vi "TUNA RT main.vi"() -> ()   [LabVIEW 2014]
uses:
  <vilib>/myRIO/Instrument Drivers/Onboard IO/AI/AI.lvlib
  <vilib>/myRIO/Common/Instrument Driver Framework/Utilities/typedefs/Analog Scaling Constants.ctl
  <vilib>/myRIO/Common/Instrument Driver Framework/Utilities/typedefs/Analog Scaling Constants List.ctl
  <vilib>/myRIO/Common/Instrument Driver Framework/myRIO v1.0/AI/typedefs/AI Channels Enum.ctl
  <vilib>/myRIO/Common/Instrument Driver Framework/myRIO v1.0/AI/typedefs/AI Channels List.ctl
  <vilib>/myRIO/Common/Instrument Driver Framework/Utilities/typedefs/Generic FPGA Reference.ctl
  <vilib>/myRIO/Common/Instrument Driver Framework/Utilities/typedefs/myRIO v1.0 Reference.ctl
  <vilib>/myRIO/Common/Instrument Driver Framework/Utilities/typedefs/Hardware Version Enum.ctl
  <vilib>/myRIO/Common/Instrument Driver Framework/Utilities/typedefs/myRIO Generic Hardware Reference.ctl
  <vilib>/myRIO/Instrument Drivers/Onboard IO/AI/typedefs/AI Reference.ctl
  <vilib>/userdefined/High Color/nirio_resource_hc.ctl
  <vilib>/myRIO/Instrument Drivers/Onboard IO/AI/vis/myRIO AI Open.xnode
  <vilib>/myRIO/Common/Instrument Driver Framework/myRIO v1.0/DIO/typedefs/DIO Channels Enum.ctl
  <vilib>/myRIO/Common/Instrument Driver Framework/myRIO v1.0/DIO/typedefs/DIO Channels List.ctl
  <vilib>/myRIO/Instrument Drivers/Onboard IO/DIO/typedefs/DIO Reference.ctl
  <vilib>/myRIO/Instrument Drivers/Onboard IO/DIO/DIO.lvlib
  <vilib>/myRIO/Instrument Drivers/Onboard IO/DIO/vis/myRIO DIO Open.xnode
  <vilib>/myRIO/Instrument Drivers/Onboard IO/PWM/typedefs/PWM Configuration.ctl
  <vilib>/myRIO/Instrument Drivers/Onboard IO/PWM/PWM.lvlib
  <vilib>/myRIO/Common/Instrument Driver Framework/myRIO v1.0/PWM/typedefs/PWM Channels Enum.ctl
  <vilib>/myRIO/Instrument Drivers/Onboard IO/PWM/typedefs/PWM Reference.ctl
  <vilib>/myRIO/Instrument Drivers/Onboard IO/PWM/vis/myRIO PWM Open.xnode
  <vilib>/myRIO/Common/Instrument Driver Framework/myRIO v1.0/PWM/vis/myRIO v1.1 Open PWM.vi
  <vilib>/myRIO/Common/Instrument Driver Framework/myRIO v1.0/AI/vis/myRIO v1.1 Open AI.vi
  <vilib>/myRIO/Common/Instrument Driver Framework/myRIO v1.0/DIO/vis/myRIO v1.1 Open DIO.vi
  <vilib>/Instr/_visa.llb/VISA Flush IO Buffer Mask.ctl
panel:
  in  "LHEADING":dbl
  in  "LSPEED":dbl
  in  "LTAIL PERIOD":dbl
  in  "Tab Control":T1(tab)
  in  "MHeading":dbl(slide) scale=0.0005..0.0025 scale format="%_1f"
  in  "MSpeed":dbl(slide) scale=0.0005..0.0025 scale format="%#.1g"
  out "GLED":bool
  out "BLED":bool
  out "RLED":bool
  in  "stop":bool
  out "Midbrain?":bool
  out "Heading":dbl(knob) min=-45.0 max=45.0 step=1.0 scale=-45.0..45.0
  out "Speed":dbl(knob) min=-9.0 max=9.0 step=1.0 scale=-50.0..50.0
  out "Hindbrain?":bool
  out "Forebrain?":bool
  out "Battery Dead?":bool
  out "Complete?":bool=TRUE
  out "Arbiter Graph":cluster{dbl, dbl, dbl[]}(graph)
  out "GPS Time Out?":bool
  in  "Run?":bool
  in  "Manual?":bool
  out "Camera Data":T2(array[cluster])
  out "Boat Status":T3={"GPS"={"X pos"=0, "Y pos"=0, "Heading"=0.0}, "IR Sensors"=[{"Name"="Bow", "Angle"=0.0, "Distance"=0.0}], "MOT BAT"=7.2, "RIO BAT"=7.2}
  out "Act Com":T4
  out "Forebrain ACT":dbl[](array[numeric])
  out "IR Sensors":T5(array[cluster])
  out "GPS":cluster{"X pos":i32, "Y pos":i32, "Heading":dbl}
  out "RED LED":bool
  out "GREEN LED":bool
  out "BLUE LED":bool
  in  "MDF":T6(array[cluster])=[{"Type"=enum."Start", "X"=250, "Y"=250, "Speed"=0, "Behaviors"=enum."Open Water Transit"}, {"Type"=enum."Waypoint", "X"=400, "Y"=100, "Speed"=20, "Behaviors"=enum."P-Wall Follow"}, {"Type"=enum."Waypoint", "X"=250, "Y"=250, "Speed"=20, "Behaviors"=enum."Open Water Transit"}, {"Type"=enum."Waypoint", "X"=250, "Y"=400, "Speed"=20, "Behaviors"=enum."Open Water Transit"}, {"Type"=enum."Waypoint", "X"=100, "Y"=400, "Speed"=20, "Behaviors"=enum."Open Water Transit"}, {"Type"=enum."End", "X"=250, "Y"=250, "Speed"=0, "Behaviors"=enum."Open Water Transit"}]
  in  "TUNA\nTAG":string="C"
  in  "GPS\nerror in":errorcluster
  in  "GPS\nVISA resource name":refnum<visa-resource-name>="ASRL2::INSTR"
  in  "Comms\nVISA resource name":refnum<visa-resource-name>="ASRL1::INSTR"
  in  "Comms\nerror in":errorcluster
  in  "TAIL PERIOD":dbl
  out "Invalid Pos?":bool
  out "error out":errorcluster
  out "Forebrain Comd":T7
  out "Debug IR \nRaw Readings":T5(array[cluster])
  out "Comms\nHandshake?":bool
  out "GPS \nHandshake?":bool
  out "LOOP COUNT":dbl
  out "size(s)":i32
  out "MDF Active":T6(array[cluster])
  # "To start the Tug, press the \">\" key in the tool bar.\n\nPress the Run? control to start the Mission.\n\nWhen complete the Complete? indicator will light.\n\nIf the Run? is not pressed again, the mission will start again.\n\nAlways press the STOP button to end the operation!!!!!!!!!!!!!"
  # "Press the Manual? button to control\nthe Tug from the sliders"
  # "Stuck indicates that\nthe boat is not moving."
  # "Enter the Letter\nof  your Tug"
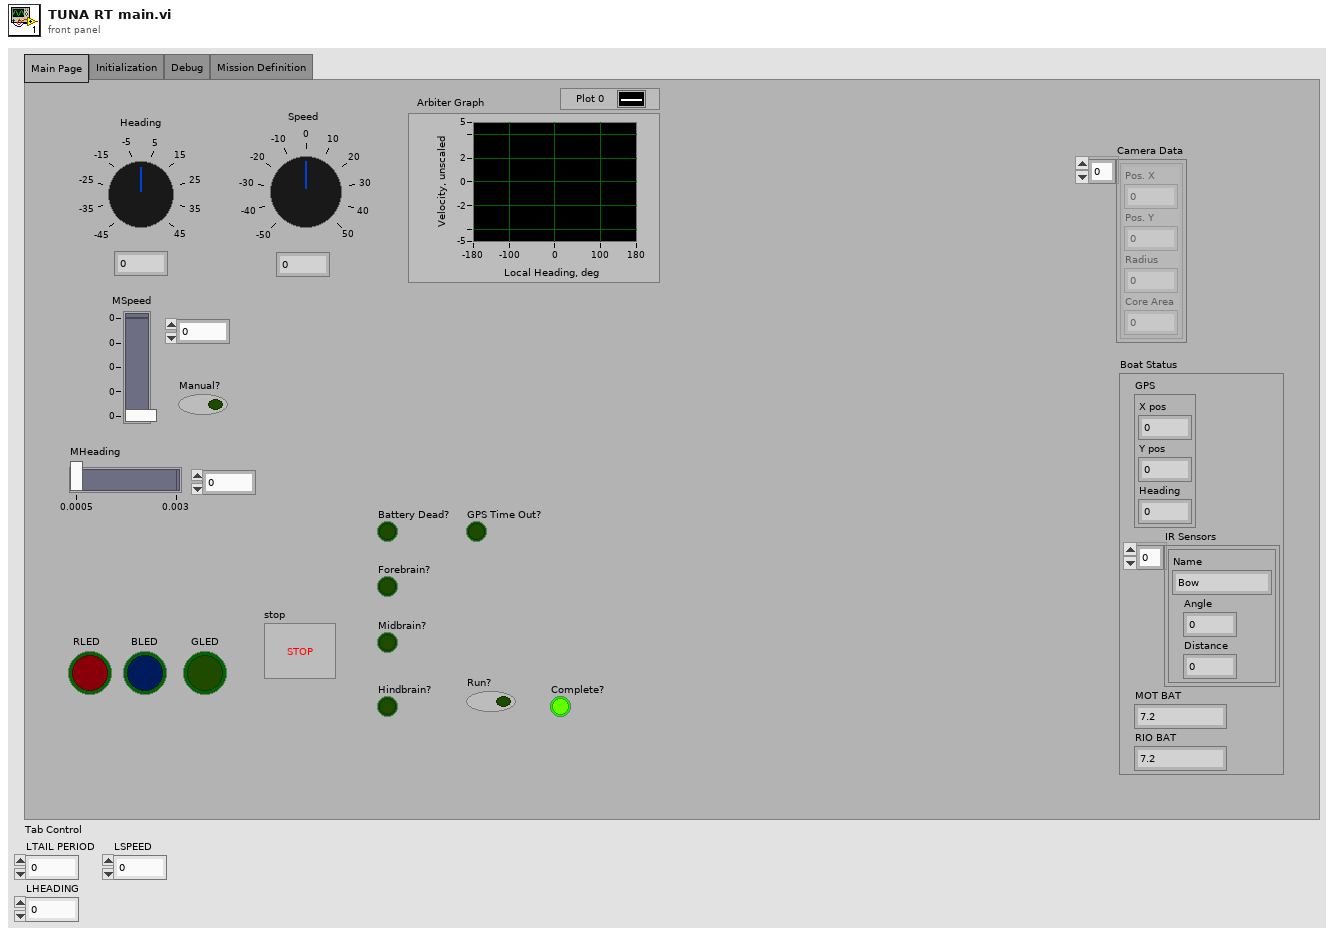
[diagram p1: front panel]
types:
  T1 = enum32{"Main Page", "Initialization", "Debug", "Mission Definition"}
  T2 = cluster{"Pos. X":i32, "Pos. Y":i32, "Radius":i32, "Core Area":i32}[]
  T3 = cluster{"GPS":cluster{"X pos":i32, "Y pos":i32, "Heading":dbl}, "IR Sensors":cluster{"Name":string, "Angle":dbl, "Distance":dbl}[], "MOT BAT":dbl, "RIO BAT":dbl}
  T4 = cluster{"Desired Local\nHeading":dbl, "Desired\nSpeed":dbl}
  T5 = cluster{"Name":string, "Angle":dbl, "Distance":dbl}[]
  T6 = cluster{"Type":enum16{"Start", "Waypoint", "End"}, "X":i32, "Y":i32, "Speed":i32, "Behaviors":enum16{"Open Water Transit", "P-Wall Follow", "S-Wall Follow", "Dock"}}[]
  T7 = cluster{"Behaviors":enum16{"Open Water Transit", "P-Wall Follow", "S-Wall Follow", "Dock"}, "Behavior\nVelocity":dbl}
  T8 = typedef "nirio_resource_hc.ctl" = tag
  T9 = typedef "Hardware Version Enum.ctl" = enum16{"Unknown", "myRIO-1900", "myRIO-1950"}
  T10 = enum16{"Open Water Transit", "P-Wall Follow", "S-Wall Follow", "Dock"}
  T11 = typedef "PWM.lvlib/PWM Reference.ctl" = cluster{"myRIO Reference":T12, "PWM Channels Enum":T15, "PWM Configuration":T16}
  T12 = typedef "myRIO Generic Hardware Reference.ctl" = cluster{"myRIO Model":T9, "myRIO Hardware Reference":T13}
  T13 = typedef "myRIO v1.0 Reference.ctl" = cluster{"Generic FPGA Reference":T14, "Allow multiple opens":bool}
  T14 = typedef "Generic FPGA Reference.ctl" = refnum<k20>
  T15 = typedef "PWM Channels Enum.ctl" = enum16{"Not Connected", "C/PWM0", "C/PWM1", "A/PWM0", "A/PWM1", "A/PWM2", "B/PWM0", "B/PWM1", "B/PWM2"}
  T16 = typedef "PWM.lvlib/PWM Configuration.ctl" = cluster{"Frequency":dbl, "Duty Cycle":dbl}
  T17 = typedef "DIO.lvlib/DIO Reference.ctl" = cluster{"myRIO Reference":T12, "DIO Channels List":T18}
  T18 = typedef "DIO Channels List.ctl" = T19[]
  T19 = typedef "DIO Channels Enum.ctl" = enum16{"Not Connected", "C/DIO0", "C/DIO1", "C/DIO2", "C/DIO3", "C/DIO4", "C/DIO5", "C/DIO6", "C/DIO7", "A/DIO0", "A/DIO1", "A/DIO2", "A/DIO3", "A/DIO4", "A/DIO5", "A/DIO6", "A/DIO7", "A/DIO8", "A/DIO9", "A/DIO10", "A/DIO11", "A/DIO12", "A/DIO13", "A/DIO14", "A/DIO15", "B/DIO0", "B/DIO1", "B/DIO2", "B/DIO3", "B/DIO4", "B/DIO5", "B/DIO6", "B/DIO7", "B/DIO8", "B/DIO9", "B/DIO10", "B/DIO11", "B/DIO12", "B/DIO13", "B/DIO14", "B/DIO15", "LED0", "LED1", "LED2", "LED3", "Button0"}
  T20 = typedef "AI.lvlib/AI Reference.ctl" = cluster{"myRIO Reference":T12, "AI Channels List":T21, "AI Scaling Constants List":T23}
  T21 = typedef "AI Channels List.ctl" = T22[]
  T22 = typedef "AI Channels Enum.ctl" = enum16{"Not Connected", "AudioIn/Left", "AudioIn/Right", "C/AI0", "C/AI1", "A/AI0", "A/AI1", "A/AI2", "A/AI3", "B/AI0", "B/AI1", "B/AI2", "B/AI3"}
  T23 = typedef "Analog Scaling Constants List.ctl" = T24[]
  T24 = typedef "Analog Scaling Constants.ctl" = cluster{"LSB Weight (Volts)":dbl, "Offset (Volts)":dbl, "Signed?":bool}
  T25 = cluster{"Obs Avoid Array":dbl[], "P-Wall Array":dbl[], "S-Wall Array":dbl[], "Unstuck Array":dbl[]}
  T26 = typedef "VISA Flush IO Buffer Mask.ctl" = u16
  T27 = cluster{"Behaviors":enum16{"Open Water Transit", "P-Wall Follow", "S-Wall Follow", "Dock"}, dbl}
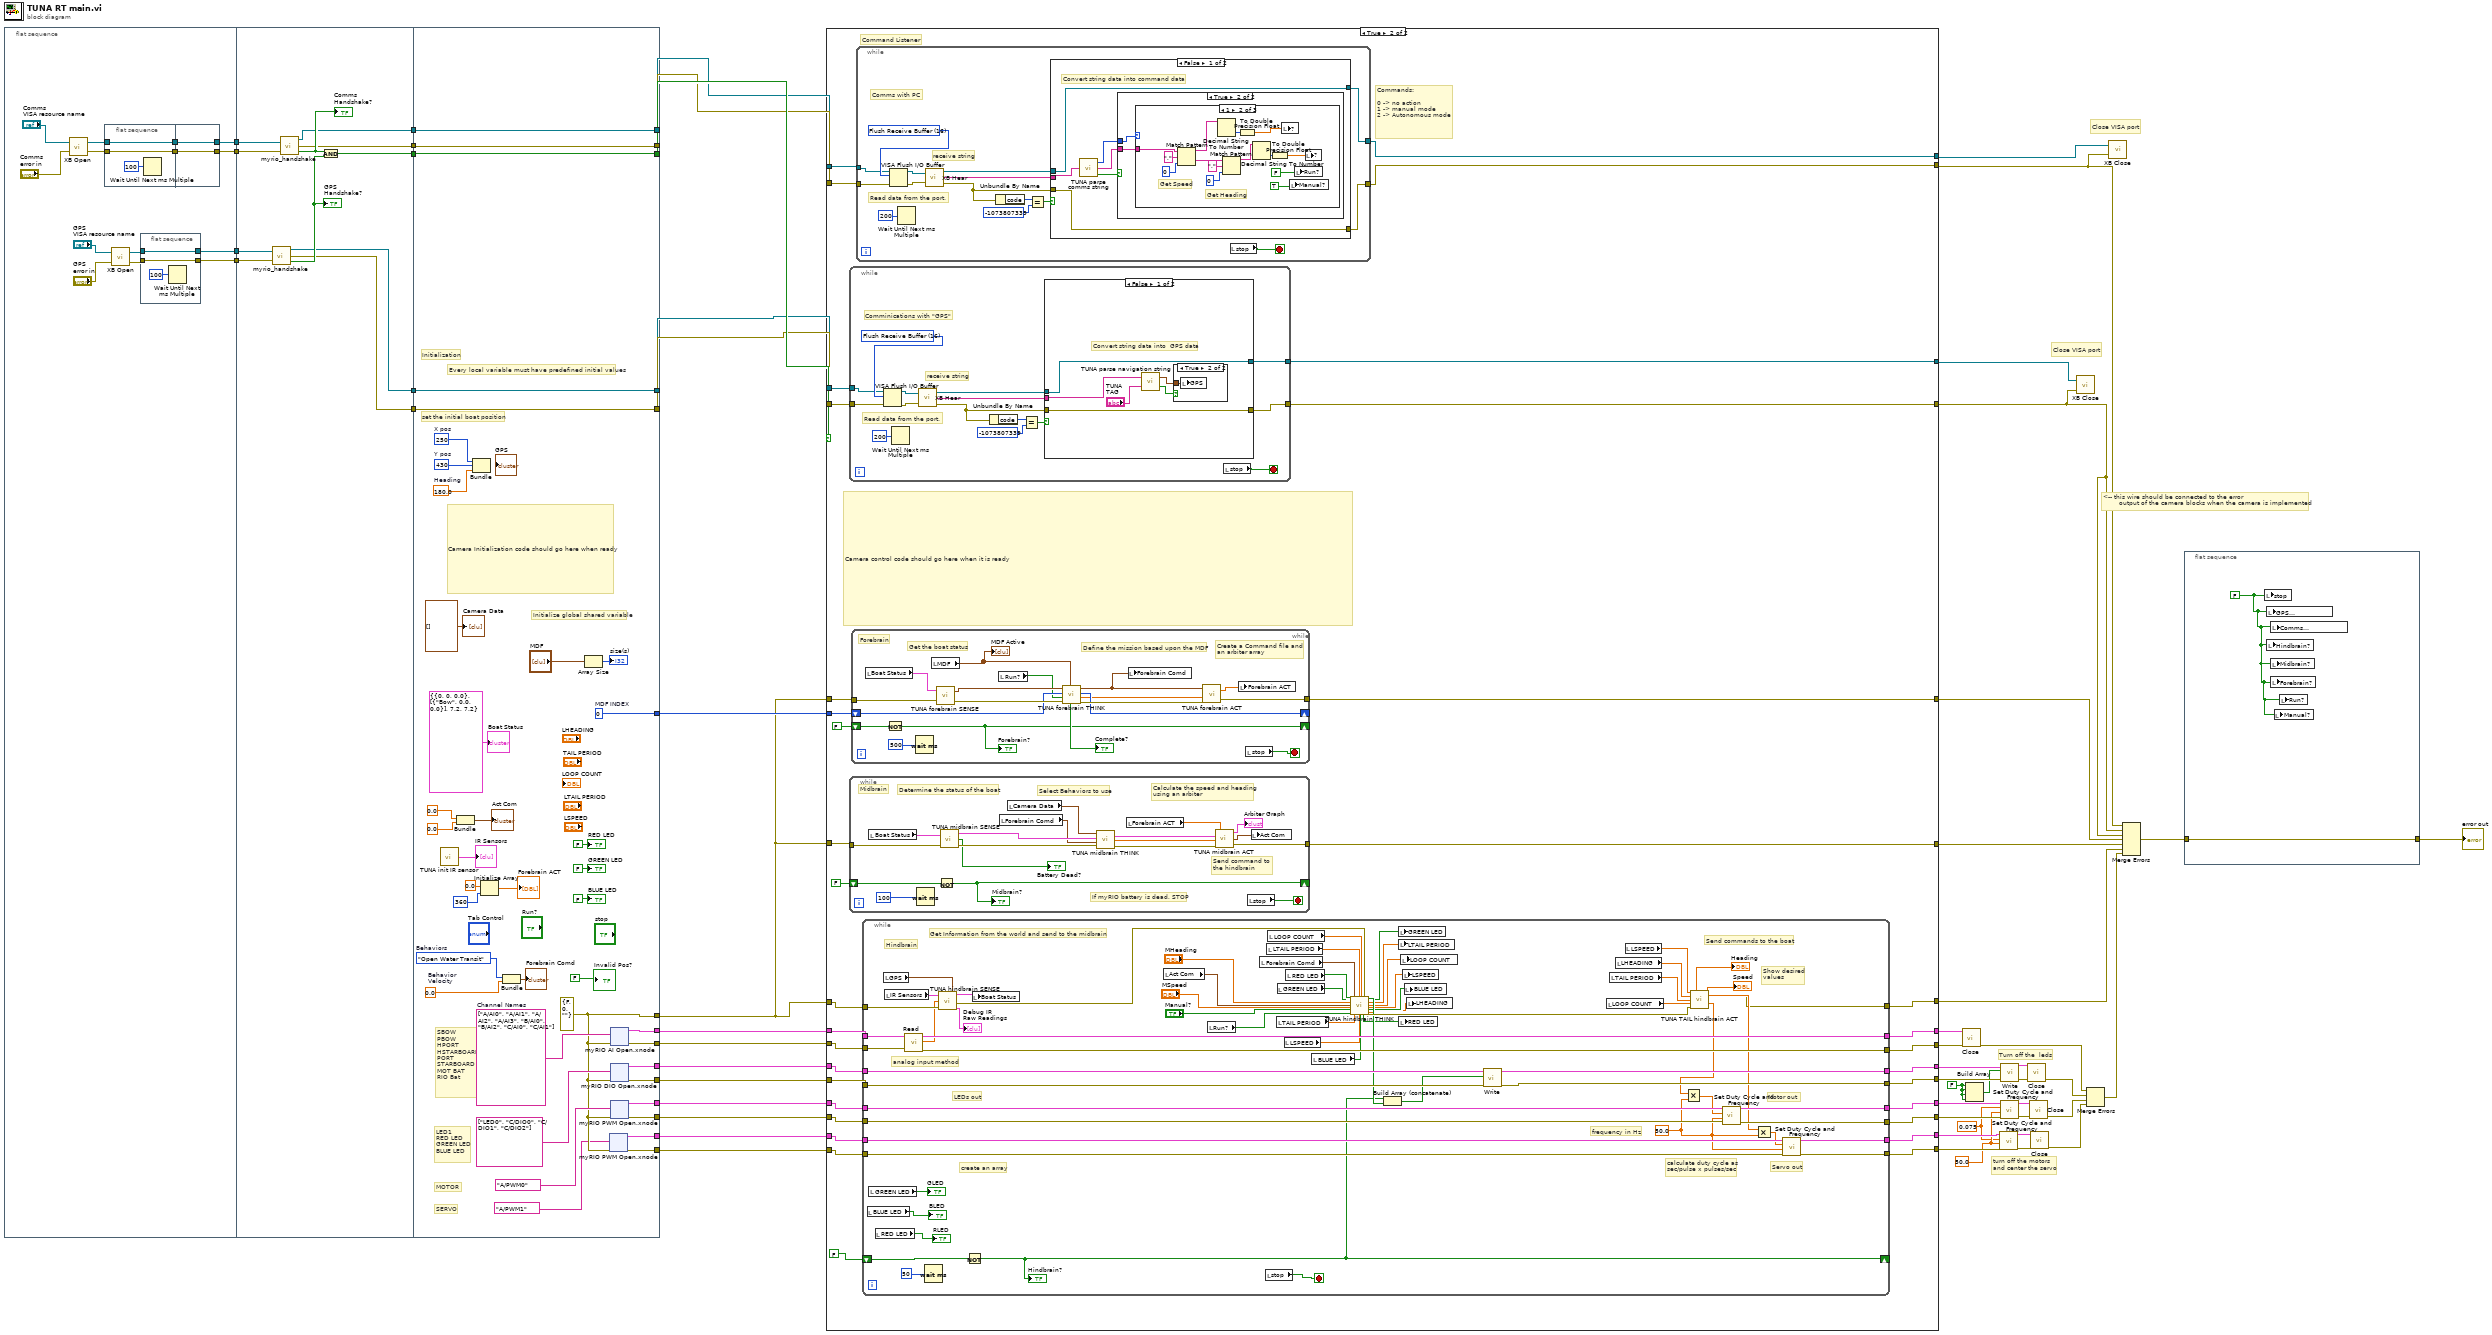
[diagram p0: block diagram]
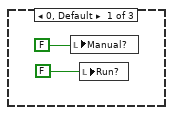
[diagram p4: hidden frame]
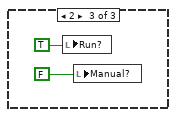
[diagram p5: hidden frame]
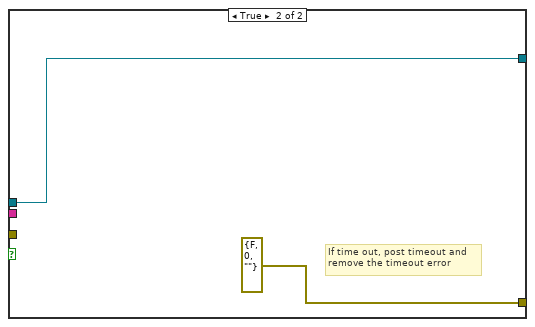
[diagram p6: hidden frame]
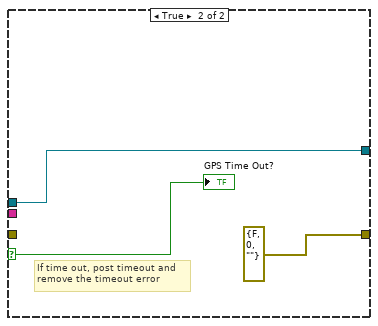
[diagram p8: hidden frame]
diagram:
  w23 = 0.075
  w22 = FALSE
  w24 = 50.0
  # "Close VISA port"
  # "<-- this wire should be connected to the error\n        output of the camera blocks when the camera is implemented"
  # "Close VISA port"
  # "Turn off the  leds"
  # "turn off the motors\nand center the servo"
  n1 = flat-sequence {
    tunnel: [w60] -> w10
    tunnel: [w59] -> w9
    tunnel: [w58] -> w8
    tunnel: [w57] -> w7
    tunnel: [w87] -> w11
    tunnel: w10 -> [w86]
    tunnel: w9 -> [w85]
    tunnel: w8 -> [w84]
    tunnel: w7 -> [w83]
    tunnel: [w82] -> w6
    tunnel: [w81] -> w5
    tunnel: [w80] -> w4
    tunnel: [w79] -> w3
    tunnel: w11 -> [w94]
    tunnel: w6 -> [w93]
    tunnel: w5 -> [w92]
    tunnel: w4 -> [w91]
    tunnel: w3 -> [w90]
    tunnel: [w106] -> w17
    tunnel: [w121] -> w53
    tunnel: [w114] -> w52
    tunnel: [w113] -> w51
    tunnel: [w111] -> w47
    tunnel: [w110] -> w48
    tunnel: [w108] -> w46
    tunnel: [w107] -> w45
    tunnel: [w104] -> w44
    tunnel: [w103] -> w43
    tunnel: [w94] -> w21
    tunnel: [w93] -> w19
    tunnel: [w92] -> w20
    tunnel: [w91] -> w14
    tunnel: [w90] -> w15
    frame #0 {
      n2 = call "XB Open.vi"("error in (no error)"="Comms\nerror in", "VISA resource name"="Comms\nVISA resource name") -> ("error out"=w68:errorcluster, "VISA resource name out"=w67:refnum<visa-resource-name>)
      n3 = flat-sequence {
        tunnel: w67 -> [w74]
        tunnel: w68 -> [w75]
        tunnel: [w75] -> w70
        tunnel: [w74] -> w69
        tunnel: [w77] -> w60
        tunnel: [w78] -> w59
        tunnel: w70 -> [w78]
        tunnel: w69 -> [w77]
        frame #0 {
          n4 = Wait Until Next ms Multiple(millisecond multiple=u32 100) -> ()  [unwired: 1 out]
        }
        frame #1 {
        }
      }
      n5 = call "XB Open.vi"("error in (no error)"="GPS\nerror in", "VISA resource name"="GPS\nVISA resource name") -> ("error out"=w63:errorcluster, "VISA resource name out"=w64:refnum<visa-resource-name>)
      n6 = flat-sequence {
        tunnel: w64 -> [w71]
        tunnel: w63 -> [w72]
        tunnel: [w72] -> w57
        tunnel: [w71] -> w58
        frame #0 {
          n7 = Wait Until Next ms Multiple(millisecond multiple=u32 100) -> ()  [unwired: 1 out]
        }
      }
    }
    frame #1 {
      n8 = call "myrio_handshake.vi"("VISA resource name"=w84, "error in"=w83) -> ("VISA resource name out"=w82:refnum<visa-resource-name>, "error out"=w81:errorcluster, "All Clear \nfrom PC?"=w89:bool)
      "GPS \nHandshake?" <- w89
      n9 = call "myrio_handshake.vi"("VISA resource name"=w86, "error in"=w85) -> ("VISA resource name out"=w80:refnum<visa-resource-name>, "error out"=w79:errorcluster, "All Clear \nfrom PC?"=w88:bool)
      "Comms\nHandshake?" <- w88
      n10 = And(x=w88, y=w89) -> (x .and. y?=w87:bool)
    }
    frame #2 {
      w115 = tag[] ["A/AI0", "A/AI1", "A/AI2", "A/AI3", "B/AI0", "B/AI2", "C/AI0", "C/AI1"]  # Channel Names
      w116 = 430  # Y pos
      w117 = 250  # X pos
      w118 = 180.0  # Heading
      w106 = errorcluster {"status"=FALSE, "code"=0, "source"=""} ("error out")
      w121 = 0  # MDF INDEX
      w125 = 0.0  # Behavior Velocity
      w120 = T10."Open Water Transit"  # Behaviors
      # "Camera Initialization code should go here when ready"
      # "Initialize global shared variable"
      # "LED1\nRED LED\nGREEN LED\nBLUE LED"
      # "SERVO"
      # "MOTOR"
      # "SBOW\nPBOW\nHPORT\nHSTARBOARD\nPORT\nSTARBOARD\nMOT BAT\nRIO Bat"
      # "set the initial boat position"
      # "Every local variable must have predefined initial values"
      # "Initialization"
      n11 = call "TUNA init IR sensor.vi"() -> ("IR Sensors"=→"IR Sensors":T5)  [unwired: 1 in]
      n12 = Bundle(0.0, 0.0) -> (→"Act Com":cluster{dbl, dbl})  [unwired: 1 in]
      n13 = Bundle("X pos"=w117, "Y pos"=w116, "Heading"=w118) -> ()  [unwired: 1 in, 1 out]
      n14 = Initialize Array(0.0 ("element"), 360 ("dimension size")) -> (→"Forebrain ACT":dbl[])
      n15 = Bundle("Behaviors"=w120, "Behavior\nVelocity"=w125) -> (→"Forebrain Comd":T7)  [unwired: 1 in]
      n16 = Array Size(array="MDF") -> (size(s)=→"size(s)":i32)
      n17 = xnode "myRIO PWM Open.xnode"("error in (no error)"=w106, "Channel Name"=tag "A/PWM1") -> ("error out"=w104:errorcluster, "PWM Ref Out"=w103:T11)  [unwired: 1 in]
      n18 = xnode "myRIO DIO Open.xnode"("error in (no error)"=w106, "Channel Names"=tag[] ["LED0", "C/DIO0", "C/DIO1", "C/DIO2"]) -> ("error out"=w111:errorcluster, "DIO Ref Out"=w110:T17)  [unwired: 1 in]
      n19 = xnode "myRIO PWM Open.xnode"("error in (no error)"=w106, "Channel Name"=tag "A/PWM0") -> ("error out"=w108:errorcluster, "PWM Ref Out"=w107:T11)  [unwired: 1 in]
      n20 = xnode "myRIO AI Open.xnode"("error in (no error)"=w106, "Channel Names"=w115) -> ("error out"=w114:errorcluster, "AI Ref Out"=w113:T20)  [unwired: 1 in]
      "Invalid Pos?" <- FALSE
      "RED LED" <- FALSE ("RED LED")
      "GREEN LED" <- FALSE ("GREEN LED")
      "BLUE LED" <- FALSE ("WHITE LED")
      "Camera Data" <- T2 [] ("Camera Data")
      "Boat Status" <- T3 {"GPS"={"X pos"=0, "Y pos"=0, "Heading"=0.0}, "IR Sensors"=[{"Name"="Bow", "Angle"=0.0, "Distance"=0.0}], "MOT BAT"=7.2, "RIO BAT"=7.2} ("Boat Status 2")
    }
  }
  n21 = case shown="True" w21 {
    tunnel: [w199 w241] -> w56
    tunnel: [w199 w240] -> w55
    tunnel: w17 -> [w199 w238]
    tunnel: [w199 w236] -> w54
    tunnel: w53 -> [_ w235]
    tunnel: [w200 w216] -> w16
    tunnel: w52 -> [w202 w234]
    tunnel: w51 -> [w201 w233]
    tunnel: [w202 w232] -> w50
    tunnel: [w201 w231] -> w49
    tunnel: w48 -> [w203 w230]
    tunnel: w47 -> [w204 w229]
    tunnel: w46 -> [w206 w228]
    tunnel: w45 -> [w205 w227]
    tunnel: w44 -> [w208 w226]
    tunnel: w43 -> [w207 w225]
    tunnel: [w208 w224] -> w42
    tunnel: [w207 w223] -> w40
    tunnel: [w206 w222] -> w38
    tunnel: [w205 w221] -> w35
    tunnel: [w204 w220] -> w29
    tunnel: [w203 w219] -> w26
    tunnel: w20 -> [w200 w218]
    tunnel: w19 -> [w198 w217]
    tunnel: [w198 w215] -> w18
    tunnel: w17 -> [_ w213]
    tunnel: w17 -> [_ w214]
    tunnel: w15 -> [w196 w211]
    tunnel: w14 -> [w197 w212]
    tunnel: [w197 w210] -> w13
    tunnel: [w196 w209] -> w12
    frame False {
    }
    frame True {
      # "Commands:\n\n0 -> no action\n1 -> manual mode\n2 -> Autonomous mode"
      # "Command Listener"
      # "Camera control code should go here when it is ready"
      n22 = while {
        shift-right: [w399] -> _
        shift-left: FALSE -> [w410]
        tunnel: w213 -> [w409]
        tunnel: [w403] -> w240
        stop <- w411 stop-if-true
        # "If myRIO battery is dead, STOP"
        # "Send command to \nthe hindbrain"
        # "Calculate the speed and heading\nusing an arbiter"
        # "Select Behaviors to use"
        # "Determine the status of the boat"
        # "Midbrain"
        n23 = local read "Boat Status"() -> (w394:T3)
        n24 = Wait (ms)(milliseconds to wait=u32 100) -> ()  [unwired: 1 out]
        n25 = Not(x=w410) -> (.not. x?=w399:bool)
        "Midbrain?" <- w399
        n26 = call "TUNA midbrain SENSE.vi"("Boat Status"=w394, "error in"=w409) -> ("IR Sensors"=w397:T5, "Battery\nDead?"=→"Battery Dead?":bool, "error out"=w407:errorcluster)
        n27 = local read "Forebrain Comd"() -> (w396:T7)
        n28 = local read "Camera Data"() -> (w395:T2)
        n29 = call "TUNA midbrain THINK.vi"("error in"=w407, "Forebrain Comd"=w396, "IR Sensors"=w397, "Camera Data"=w395) -> ("error out"=w406:errorcluster, "Behavior\nVelocity OUT"=w401:dbl, "Behavior arrays"=w404:T25)
        n30 = local read "Forebrain ACT"() -> (w402:dbl[])
        n31 = call "TUNA midbrain ACT.vi"("error in"=w406, "Behavior\nVelocity"=w401, "Behavior arrays"=w404, "Forebrain ACT"=w402) -> ("error out"=w403:errorcluster, "Act Com"=w408:T4, "Waveform Graph"=→"Arbiter Graph":cluster{dbl, dbl, dbl[]})
        n32 = local read "stop"() -> (w411:bool)
        n33 = local write "Act Com"(w408) -> ()
      }
      n34 = while {
        tunnel: w218 -> [w294]
        tunnel: w217 -> [w295]
        tunnel: [w291] -> w216
        tunnel: [w286] -> w215
        stop <- w297 stop-if-true
        w296 = T26 16 items=["Flush Receive Buffer"=16, "Write Transmit Buffer to Device"=32, "Flush Receive Buffer (No I/O)"=64, "Flush Transmit Buffer"=128] ("Mask")
        # "Comminications with \"GPS\""
        # "receive string"
        # "Read data from the port."
        n35 = VISA Flush I/O Buffer(VISA resource name=w295, mask (16)=w296, error in (no error)=w294) -> (VISA resource name out=w293:refnum<visa-resource-name>, error out=w292:errorcluster)
        n36 = Wait Until Next ms Multiple(millisecond multiple=u32 200) -> ()  [unwired: 1 out]
        n37 = call "XB Hear.vi"("VISA resource name"=w293, "error in (no error)"=w292) -> ("VISA resource name out"=w290:refnum<visa-resource-name>, "String Received"=w289:string, "error out"=w287:errorcluster)
        n38 = Unbundle By Name(w287) -> ("code"=w300:i32)
        n39 = Equal?(x=w300, y=-1073807339) -> (x = y?=w288:bool)
        n40 = case shown="False" w288 {
          selector: w288 -> [_ w310]
          tunnel: [w302 errorcluster {"status"=FALSE, "code"=0, "source"=""} ("error out")] -> w291
          tunnel: w290 -> [w304 w309]
          tunnel: w289 -> [w305 _]
          tunnel: [w304 w309] -> w286
          tunnel: w287 -> [w302 _]
          frame False {
            # "Convert string data into  GPS data"
            n41 = call "TUNA parse navigation string.vi"("Header"="TUNA\nTAG", "Nav String"=w305) -> ("Valid?"=w301:bool, "Output GPS"=w303:cluster{"X POS":i32, "Y POS":i32, "HEADING":dbl})
            n42 = case shown="True" w301 {
              tunnel: w303 -> [_ w307]
              frame False {
              }
              frame True {
                n43 = local write "GPS"(w307) -> ()
              }
            }
          }
          frame True {
            # "If time out, post timeout and\nremove the timeout error"
            "GPS Time Out?" <- w310
          }
        }
        n44 = local read "stop"() -> (w297:bool)
      }
      n45 = while {
        tunnel: w214 -> [w326]
        shift-right: [w314] -> _
        shift-left: FALSE -> [w315]
        tunnel: [w323] -> w236
        shift-right: [w319] -> _
        shift-left: w235 -> [w317]
        stop <- w327 stop-if-true
        # "Create a Command file and \nan arbiter array"
        # "Define the mission based upon the MDF"
        # "Get the boat status"
        # "Forebrain"
        n46 = local read "Boat Status"() -> (w321:T3)
        n47 = Not(x=w315) -> (.not. x?=w314:bool)
        "Forebrain?" <- w314
        n48 = Wait (ms)(milliseconds to wait=u32 500) -> ()  [unwired: 1 out]
        n49 = local read "MDF"() -> (w311:T6)
        "MDF Active" <- w311
        n50 = call "TUNA forebrain SENSE.vi"("error in"=w326, "Boat Status"=w321) -> ("error out"=w325:errorcluster, "GPS"=w320:cluster{"X pos":i32, "Y pos":i32, "Heading":dbl})  [unwired: 1 in]
        n51 = local read "Run?"() -> (w313:bool)
        n52 = call "TUNA forebrain THINK.vi"("MDF in"=w311, "error in"=w325, "Run?"=w313, "MDF index"=w317, "GPS"=w320) -> ("error out"=w324:errorcluster, "local Steering\nangle"=w318:dbl, "MDF Index out"=w319:i32, "Behaviors out"=w312:T27, "Complete?"=→"Complete?":bool)
        n53 = local write "Forebrain Comd"(w312) -> ()
        n54 = call "TUNA forebrain ACT.vi"("error in"=w324, "local Steering\nangle"=w318, "Behaviors in"=w312) -> ("error out"=w323:errorcluster, "Forebrain ACT"=w322:dbl[])
        n55 = local write "Forebrain ACT"(w322) -> ()
        n56 = local read "stop"() -> (w327:bool)
      }
      n57 = while {
        tunnel: w211 -> [w251]
        tunnel: w212 -> [w252]
        tunnel: [w248] -> w209
        tunnel: [w243] -> w210
        stop <- w254 stop-if-true
        w253 = T26 16 items=["Flush Receive Buffer"=16, "Write Transmit Buffer to Device"=32, "Flush Receive Buffer (No I/O)"=64, "Flush Transmit Buffer"=128] ("Mask")
        # "Comms with PC"
        # "receive string"
        # "Read data from the port."
        n58 = VISA Flush I/O Buffer(VISA resource name=w252, mask (16)=w253, error in (no error)=w251) -> (VISA resource name out=w250:refnum<visa-resource-name>, error out=w249:errorcluster)
        n59 = Wait Until Next ms Multiple(millisecond multiple=u32 200) -> ()  [unwired: 1 out]
        n60 = call "XB Hear.vi"("VISA resource name"=w250, "error in (no error)"=w249) -> ("VISA resource name out"=w247:refnum<visa-resource-name>, "String Received"=w246:string, "error out"=w244:errorcluster)
        n61 = Unbundle By Name(w244) -> ("code"=w257:i32)
        n62 = Equal?(x=w257, y=-1073807339) -> (x = y?=w245:bool)
        n63 = case shown="False" w245 {
          tunnel: [w262 errorcluster {"status"=FALSE, "code"=0, "source"=""} ("error out")] -> w248
          tunnel: w247 -> [w263 w285]
          tunnel: w246 -> [w261 _]
          tunnel: [w263 w285] -> w243
          tunnel: w244 -> [w262 _]
          frame False {
            # "Convert string data into command data"
            n64 = call "TUNA parse comms string.vi"("Nav String"=w261) -> ("Command Mode"=w258:i32, "command string"=w259:string, "Valid?"=w260:bool)
            n65 = case shown="True" w260 {
              tunnel: w259 -> [_ w264]
              tunnel: w258 -> [_ w265]
              frame False {
              }
              frame True {
                n66 = case shown="1" w265 {
                  tunnel: w264 -> [_ w274 _]
                  frame 0, Default {
                    n67 = local write "Manual?"(FALSE) -> ()
                    n68 = local write "Run?"(FALSE) -> ()
                  }
                  frame 1 {
                    # "Get Heading"
                    # "Get Speed"
                    n69 = Match Pattern(string=w274, regular expression=",", offset (0)=0) -> (before substring=w277:string, after substring=w281:string)  [unwired: 2 out]
                    n70 = Decimal String To Number(string=w277) -> (number=w270:i32)  [unwired: 2 in, 1 out]
                    n71 = Match Pattern(string=w281, regular expression=",", offset (0)=0) -> (before substring=w280:string)  [unwired: 3 out]
                    n72 = To Double Precision Float(number=w270) -> (double precision float=w269:dbl)
                    n73 = Decimal String To Number(string=w280) -> (number=w272:i32)  [unwired: 2 in, 1 out]
                    n74 = To Double Precision Float(number=w272) -> (double precision float=w271:dbl)
                    n75 = local write item#-1(w269) -> ()
                    n76 = local write "Manual?"(TRUE) -> ()
                    n77 = local write "Run?"(FALSE) -> ()
                    n78 = local write item#-1(w271) -> ()
                  }
                  frame 2 {
                    n79 = local write "Run?"(TRUE) -> ()
                    n80 = local write "Manual?"(FALSE) -> ()
                  }
                }
              }
            }
          }
          frame True {
            # "If time out, post timeout and\nremove the timeout error"
          }
        }
        n81 = local read "stop"() -> (w254:bool)
      }
      n82 = while {
        tunnel: w238 -> [w391]
        tunnel: [w346] -> w241
        shift-right: [w358] -> _
        shift-left: FALSE -> [w380]
        tunnel: w234 -> [w388]
        tunnel: w233 -> [w387]
        tunnel: [w386] -> w232
        tunnel: [w385] -> w231
        tunnel: w230 -> [w383]
        tunnel: w229 -> [w384]
        tunnel: [w382] -> w220
        tunnel: [w381] -> w219
        tunnel: w228 -> [w378]
        tunnel: w227 -> [w379]
        tunnel: [w377] -> w222
        tunnel: [w376] -> w221
        tunnel: w226 -> [w375]
        tunnel: [w374] -> w224
        tunnel: w225 -> [w373]
        tunnel: [w372] -> w223
        stop <- w393 stop-if-true
        w368 = 50.0
        # "create an array"
        # "frequency in Hz"
        # "calculate duty cycle as\nsec/pulse x pulses/sec"
        # "Show desired\nvalues"
        # "Motor out"
        # "Servo out"
        # "LEDs out"
        # "analog input method"
        # "Send commands to the boat"
        # "Get Information from the world and send to the midbrain"
        # "Hindbrain"
        n83 = local read "BLUE LED"() -> (→"BLED":bool)
        n84 = local read "GREEN LED"() -> (→"GLED":bool)
        n85 = local read "RED LED"() -> (→"RLED":bool)
        n86 = local read "GPS"() -> (w389:cluster{"X pos":i32, "Y pos":i32, "Heading":dbl})
        n87 = local read "IR Sensors"() -> (w356:T5)
        n88 = call <vilib>:"Read.vi"("error in (no error)"=w388, "AI Ref In"=w387) -> ("error out"=w386:errorcluster, "Values"=w371:dbl[], "AI Ref Out"=w385:T20)  [unwired: 7 in]
        n89 = Wait (ms)(milliseconds to wait=u32 50) -> ()  [unwired: 1 out]
        n90 = call "TUNA hindbrain SENSE.vi"("IR Sensors"=w356, "Analog Input Values"=w371, "error in"=w391, "GPS"=w389) -> ("Boat Status"=w357:T3, "error out"=w390:errorcluster, "IR Sensors 2"=→"Debug IR \nRaw Readings":T5)
        n91 = Not(x=w380) -> (.not. x?=w358:bool)
        "Hindbrain?" <- w358
        n92 = local write "Boat Status"(w357) -> ()
        n93 = local read "Act Com"() -> (w342:T4)
        n94 = local read "Run?"() -> (w347:bool)
        n95 = local read "Forebrain Comd"() -> (w355:T7)
        n96 = local read "stop"() -> (w393:bool)
        n97 = local read "LTAIL PERIOD"() -> (w344:dbl)
        n98 = local read "LOOP COUNT"() -> (w343:dbl)
        n99 = local read "TAIL PERIOD"() -> (w341:dbl)
        n100 = local read "GREEN LED"() -> (w360:bool)
        n101 = local read "LSPEED"() -> (w339:dbl)
        n102 = local read "RED LED"() -> (w361:bool)
        n103 = local read "BLUE LED"() -> (w359:bool)
        n104 = call "TUNA hindbrain THINK.vi"("RED LED"=w361, "GREEN LED"=w360, "MHeading"="MHeading", "Act Com"=w342, "MSpeed"="MSpeed", "MANUAL"="Manual?", "RUN?"=w347, "Forebrain Comd"=w355, "TAIL PERIOD"=w341, "LTAILPERIOD"=w344, "LSPEED"=w339, "LOOPCOUNT IN"=w343, "BLUE LED"=w359, "error in"=w390) -> ("RED LED OUT"=w354:bool, "LED array"=w363:bool[], "GREEN LED OUT"=w353:bool, "LTAILPERIOD OUT"=w336:dbl, "LOOPCOUNT OUT"=w340:dbl, "LSPEED OUT"=w335:dbl, "BLUE LED OUT"=w352:bool, "LHEADING"=w333:dbl, "error out"=w366:errorcluster)  [unwired: 5 in]
        n105 = Build Array (concatenate)(w358, w363) -> (w362:bool[])
        n106 = local write "GREEN LED"(w353) -> ()
        n107 = local write "LTAIL PERIOD"(w336) -> ()
        n108 = local write "RED LED"(w354) -> ()
        n109 = local write "LOOP COUNT"(w340) -> ()
        n110 = local write "LSPEED"(w335) -> ()
        n111 = local write "BLUE LED"(w352) -> ()
        n112 = local write "LHEADING"(w333) -> ()
        n113 = call <vilib>:"Write.vi"("error in (no error)"=w384, "Values"=w362, "DIO Ref In"=w383) -> ("error out"=w382:errorcluster, "DIO Ref Out"=w381:T17)  [unwired: 6 in]
        n114 = local read "LOOP COUNT"() -> (w338:dbl)
        n115 = local read "TAIL PERIOD"() -> (w337:dbl)
        n116 = local read "LHEADING"() -> (w331:dbl)
        n117 = local read "LSPEED"() -> (w332:dbl)
        n118 = call "TUNA TAIL hindbrain ACT.vi"("Speed Input"=w332, "Heading Input"=w331, "TAIL PERIOD"=w337, "LOOPCOUNT IN"=w338, "error in"=w366) -> ("Desired \nRudder"=→"Heading":dbl, "Rudder"=w369:dbl, "Desired\nSpeed"=→"Speed":dbl, "error out"=w346:errorcluster, "Desired Tail Position"=w345:dbl)  [unwired: 6 in]
        n119 = Multiply(x=w345, y=w368) -> (x*y=w370:dbl)
        n120 = call <vilib>:"Set Duty Cycle and Frequency.vi"("error in (no error)"=w378, "Frequency [Hz]"=w368, "Duty Cycle"=w370, "PWM Ref In"=w379) -> ("error out"=w377:errorcluster, "PWM Ref Out"=w376:T11)  [unwired: 5 in]
        n121 = Multiply(x=w369, y=w368) -> (x*y=w367:dbl)
        n122 = call <vilib>:"Set Duty Cycle and Frequency.vi"("error in (no error)"=w375, "Frequency [Hz]"=w368, "Duty Cycle"=w367, "PWM Ref In"=w373) -> ("error out"=w374:errorcluster, "PWM Ref Out"=w372:T11)  [unwired: 5 in]
      }
    }
  }
  n123 = call <vilib>:"Close.vi"("error in (no error)"=w50, "AI Ref In"=w49) -> ("error out"=w31:errorcluster)  [unwired: 9 in]
  n124 = Build Array(w22, w22, w22, w22) -> (w25:bool[])
  n125 = call <vilib>:"Set Duty Cycle and Frequency.vi"("error in (no error)"=w42, "Frequency [Hz]"=w24, "Duty Cycle"=w23, "PWM Ref In"=w40) -> ("error out"=w41:errorcluster, "PWM Ref Out"=w39:T11)  [unwired: 5 in]
  n126 = call <vilib>:"Set Duty Cycle and Frequency.vi"("error in (no error)"=w38, "Frequency [Hz]"=w24, "Duty Cycle"=w23, "PWM Ref In"=w35) -> ("error out"=w37:errorcluster, "PWM Ref Out"=w36:T11)  [unwired: 5 in]
  n127 = call <vilib>:"Write.vi"("error in (no error)"=w29, "Values"=w25, "DIO Ref In"=w26) -> ("error out"=w28:errorcluster, "DIO Ref Out"=w27:T17)  [unwired: 6 in]
  n128 = call <vilib>:"Close.vi"("error in (no error)"=w28, "DIO Ref In"=w27) -> ("error out"=w32:errorcluster)  [unwired: 9 in]
  n129 = call <vilib>:"Close.vi"("error in (no error)"=w37, "PWM Ref In"=w36) -> ("error out"=w33:errorcluster)  [unwired: 9 in]
  n130 = call <vilib>:"Close.vi"("error in (no error)"=w41, "PWM Ref In"=w39) -> ("error out"=w34:errorcluster)  [unwired: 9 in]
  n131 = call "XB Close.vi"("error in (no error)"=w16, "VISA resource name"=w18) -> ()
  n132 = Merge Errors(w31, w32, w33, w34) -> (w30:errorcluster)
  n133 = call "XB Close.vi"("error in (no error)"=w12, "VISA resource name"=w13) -> ()
  n134 = Merge Errors(w12, w16, w16, w54, w55, w56, w30) -> (w1:errorcluster)
  n135 = flat-sequence {
    tunnel: [w413] -> w2
    tunnel: w1 -> [w413]
    frame #0 {
      w412 = FALSE
      n136 = local write "stop"(w412) -> ()
      n137 = local write "GPS \nHandshake?"(w412) -> ()
      n138 = local write "Hindbrain?"(w412) -> ()
      n139 = local write "Comms\nHandshake?"(w412) -> ()
      n140 = local write "Midbrain?"(w412) -> ()
      n141 = local write "Forebrain?"(w412) -> ()
      n142 = local write "Manual?"(w412) -> ()
      n143 = local write "Run?"(w412) -> ()
    }
  }
  "error out" <- w2
